vi "F-test Calculator.vi"() -> ()   [LabVIEW 2021, in "Math.lvlib"]
uses:
  <vilib>/gmath/statdist.llb/F CDF.vi
  Math/Math.lvlib
  <vilib>/gmath/NI_Gmath.lvlib
panel:
  out "H1 Significance (%)":dbl format="%.2f"
  out "H0 Significance (%)":dbl format="%.2f"
  out "F-cdf(F)":dbl=0.6065306597126334
  out "error":i32
  in  "k2":i32=1
  in  "k1":i32=1
  in  "F":dbl=0.5
  # "Probability that the variance ratio will be larger than F if H0 is valid"
  # "Probability that the variance ratio will be larger than F if H1 is valid"
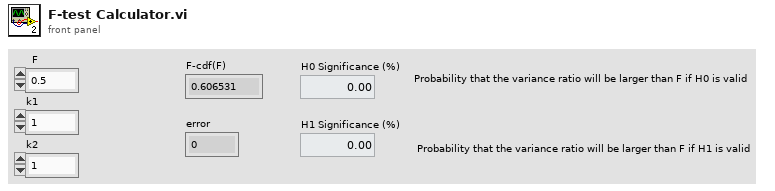
[diagram p1: front panel]
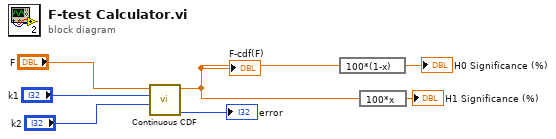
[diagram p0: block diagram]
diagram:
  n1 = call-poly <vilib>:"Continuous CDF.vi"("k2"="k2", "k1"="k1", "x"="F") -> ("error"=→"error":i32, "cdf(x)"=w2:dbl)  [unwired: 7 in]
  "F-cdf(F)" <- w2
  n2 = expression code="100*(1-x)"(w2) -> (→"H0 Significance (%)":dbl)
  n3 = expression code="100*x"(w2) -> (→"H1 Significance (%)":dbl)
